vi "Invent nestle.vi"(8 "error in (no error)":errorcluster, 10 "reemplazo":u16, 11 "Nestle Actor in":refnum<class "Nestle Actor.lvclass">) -> (0 "error out":errorcluster, 3 "Nestle Actor out":refnum<class "Nestle Actor.lvclass">)   [LabVIEW 2020, in "Nestle Actor.lvlib" / "Nestle Actor.lvclass"]
uses:
  Nestle Actor.lvclass
  Nestle Actor.lvclass/Nestle Actor.ctl
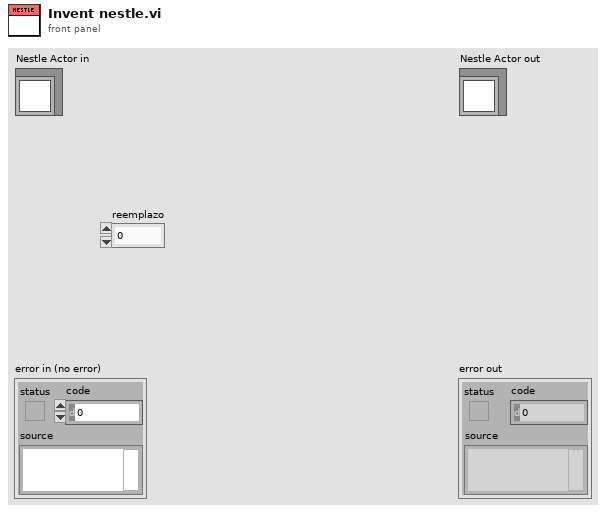
[diagram p1: front panel]
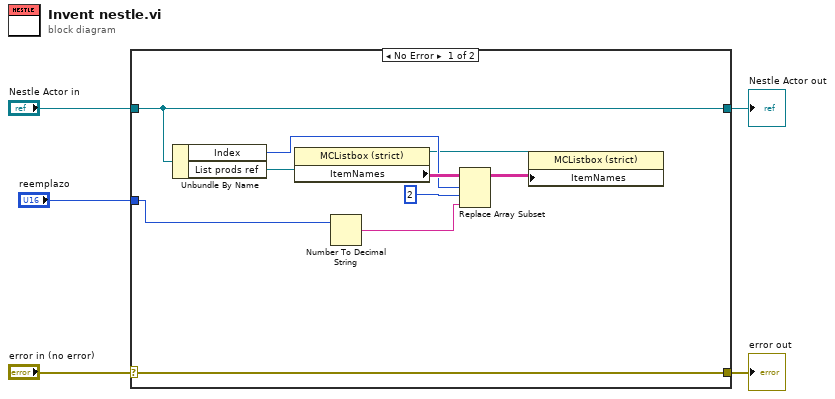
[diagram p0: block diagram]
diagram:
  n1 = case shown="No Error" "error in (no error)" {
    selector: "error in (no error)" -> [w15 w17]
    tunnel: [w15 w17] -> w4
    tunnel: [w14 w16] -> w2
    tunnel: "Nestle Actor in" -> [w14 w16]
    tunnel: "reemplazo" -> [w9 _]
    frame No Error {
      n2 = Unbundle By Name(w14) -> ("Index"=w11:u16, "List prods ref"=w13:refnum<vi>)
      n3 = property class="MCListbox (strict)"(reference=w13) -> (reference out=w7:refnum<vi>, "ItemNames"=w12:string[][])  [unwired: 1 in, 1 out]
      n4 = Number To Decimal String(number=w9) -> (decimal integer string=w8:string)  [unwired: 1 in]
      n5 = Replace Array Subset(array=w12, new element=w8, index (row)=w11, index (col)=2 ("disabled index (col)")) -> (w6:string[][])
      n6 = property class="MCListbox (strict)"(reference=w7, "ItemNames"=w6) -> ()  [unwired: 1 in, 2 out]
    }
    frame Error {
    }
  }
  "error out" <- w4
  "Nestle Actor out" <- w2
